vi "tcpGCS.vi"() -> ()   [LabVIEW 2014]
panel:
  in  "SRIC_PUSH":bool
  in  "SRIC_SSID":bool
  in  "Timer (s)":string="30"
  in  "Sync Config":bool
  in  "Password":string="pass"
  in  "Username":string="user"
  in  "Reconnect_Network":string="ubnt"
  in  "Delimiter":string="|"
  in  "File":string="msg.txt"
  in  "Directory":string="AC/"
  in  "IP Address":string="134.230.1.60"
  in  "ssid_key":string="74E87484EC"
  in  "sric_ssid":string="scrouter1"
  out "Config to Android":string
  in  "Ground Tranceiver Ip":string="192.168.1.20"
  in  "Air Tranceiver Ip":string="192.168.1.19"
  in  "Payload Ip":string="192.168.1.100"
  out "Acquiring Pictures":bool
  out "Unknown SRIC Message":string
  out "SRIC Message":string
  in  "SRIC":bool
  out "appended path":path
  out "Payload":bool
  out "Air Transceiver":bool
  out "Ground Transceiver":bool
  in  "Picture Interval":u8=3 format="%.0f seconds"
  in  "Set Picture Interval":bool
  out "connected 2":bool caption="connected"
  in  "wakeLock":bool
  in  "Rebalance":bool
  out "thing2":bool
  out "Average Time":dbl
  in  "ContinuousMode":bool
  out "thing1":bool
  out "ImageCount":u16
  out "unsigned byte array":u8[](array[numeric])
  out "Completed Images":u16[](array[numeric])
  out "OutputImages":T1(array[cluster])
  out "AverageTimePerMessage":dbl
  out "queue out":refnum<queue>
  in  "stop 2":bool
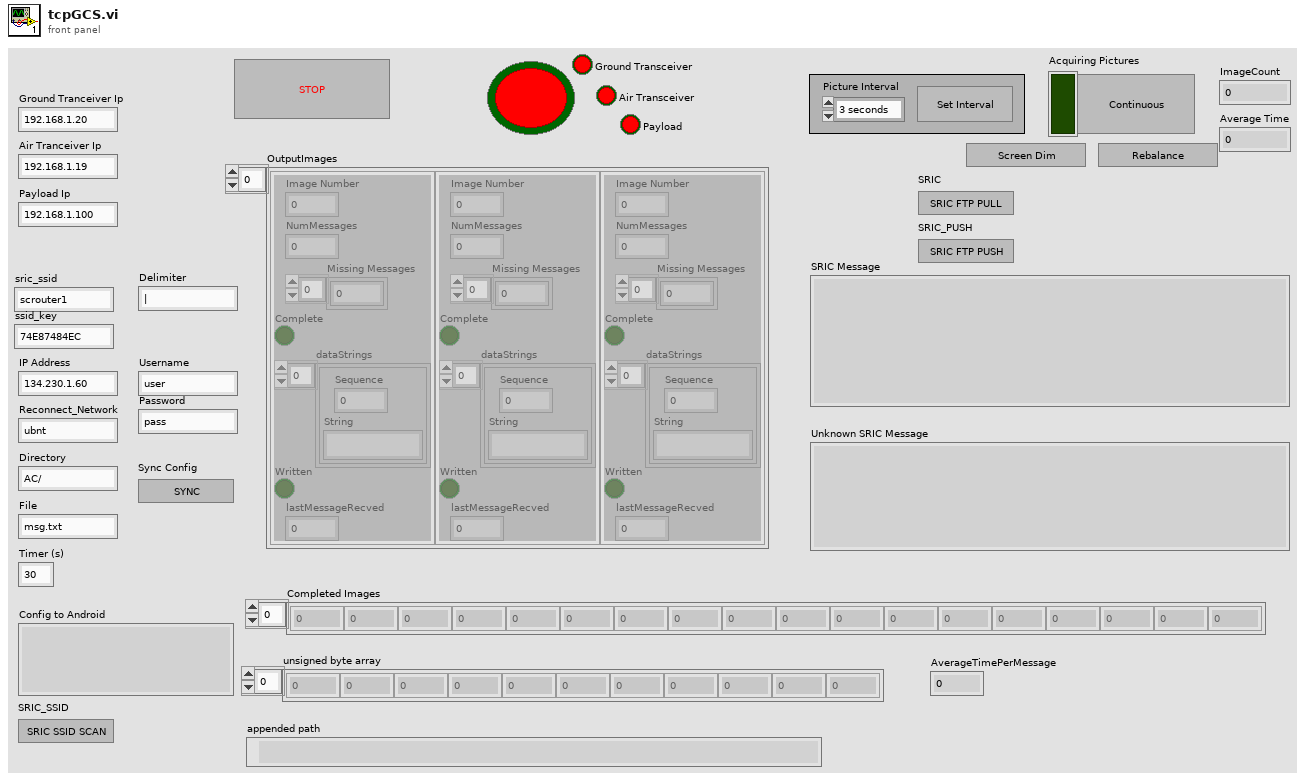
[diagram p1: front panel]
types:
  T1 = cluster{"Image Number":u16, "NumMessages":u16, "Missing Messages":u16[], "Complete":bool, "dataStrings":cluster{"Sequence":u16, "String":string}[], "Written":bool, "lastMessageRecved":u32}[]
  T2 = enum16{"Standard", "Buffered", "CRLF", "Immediate"}
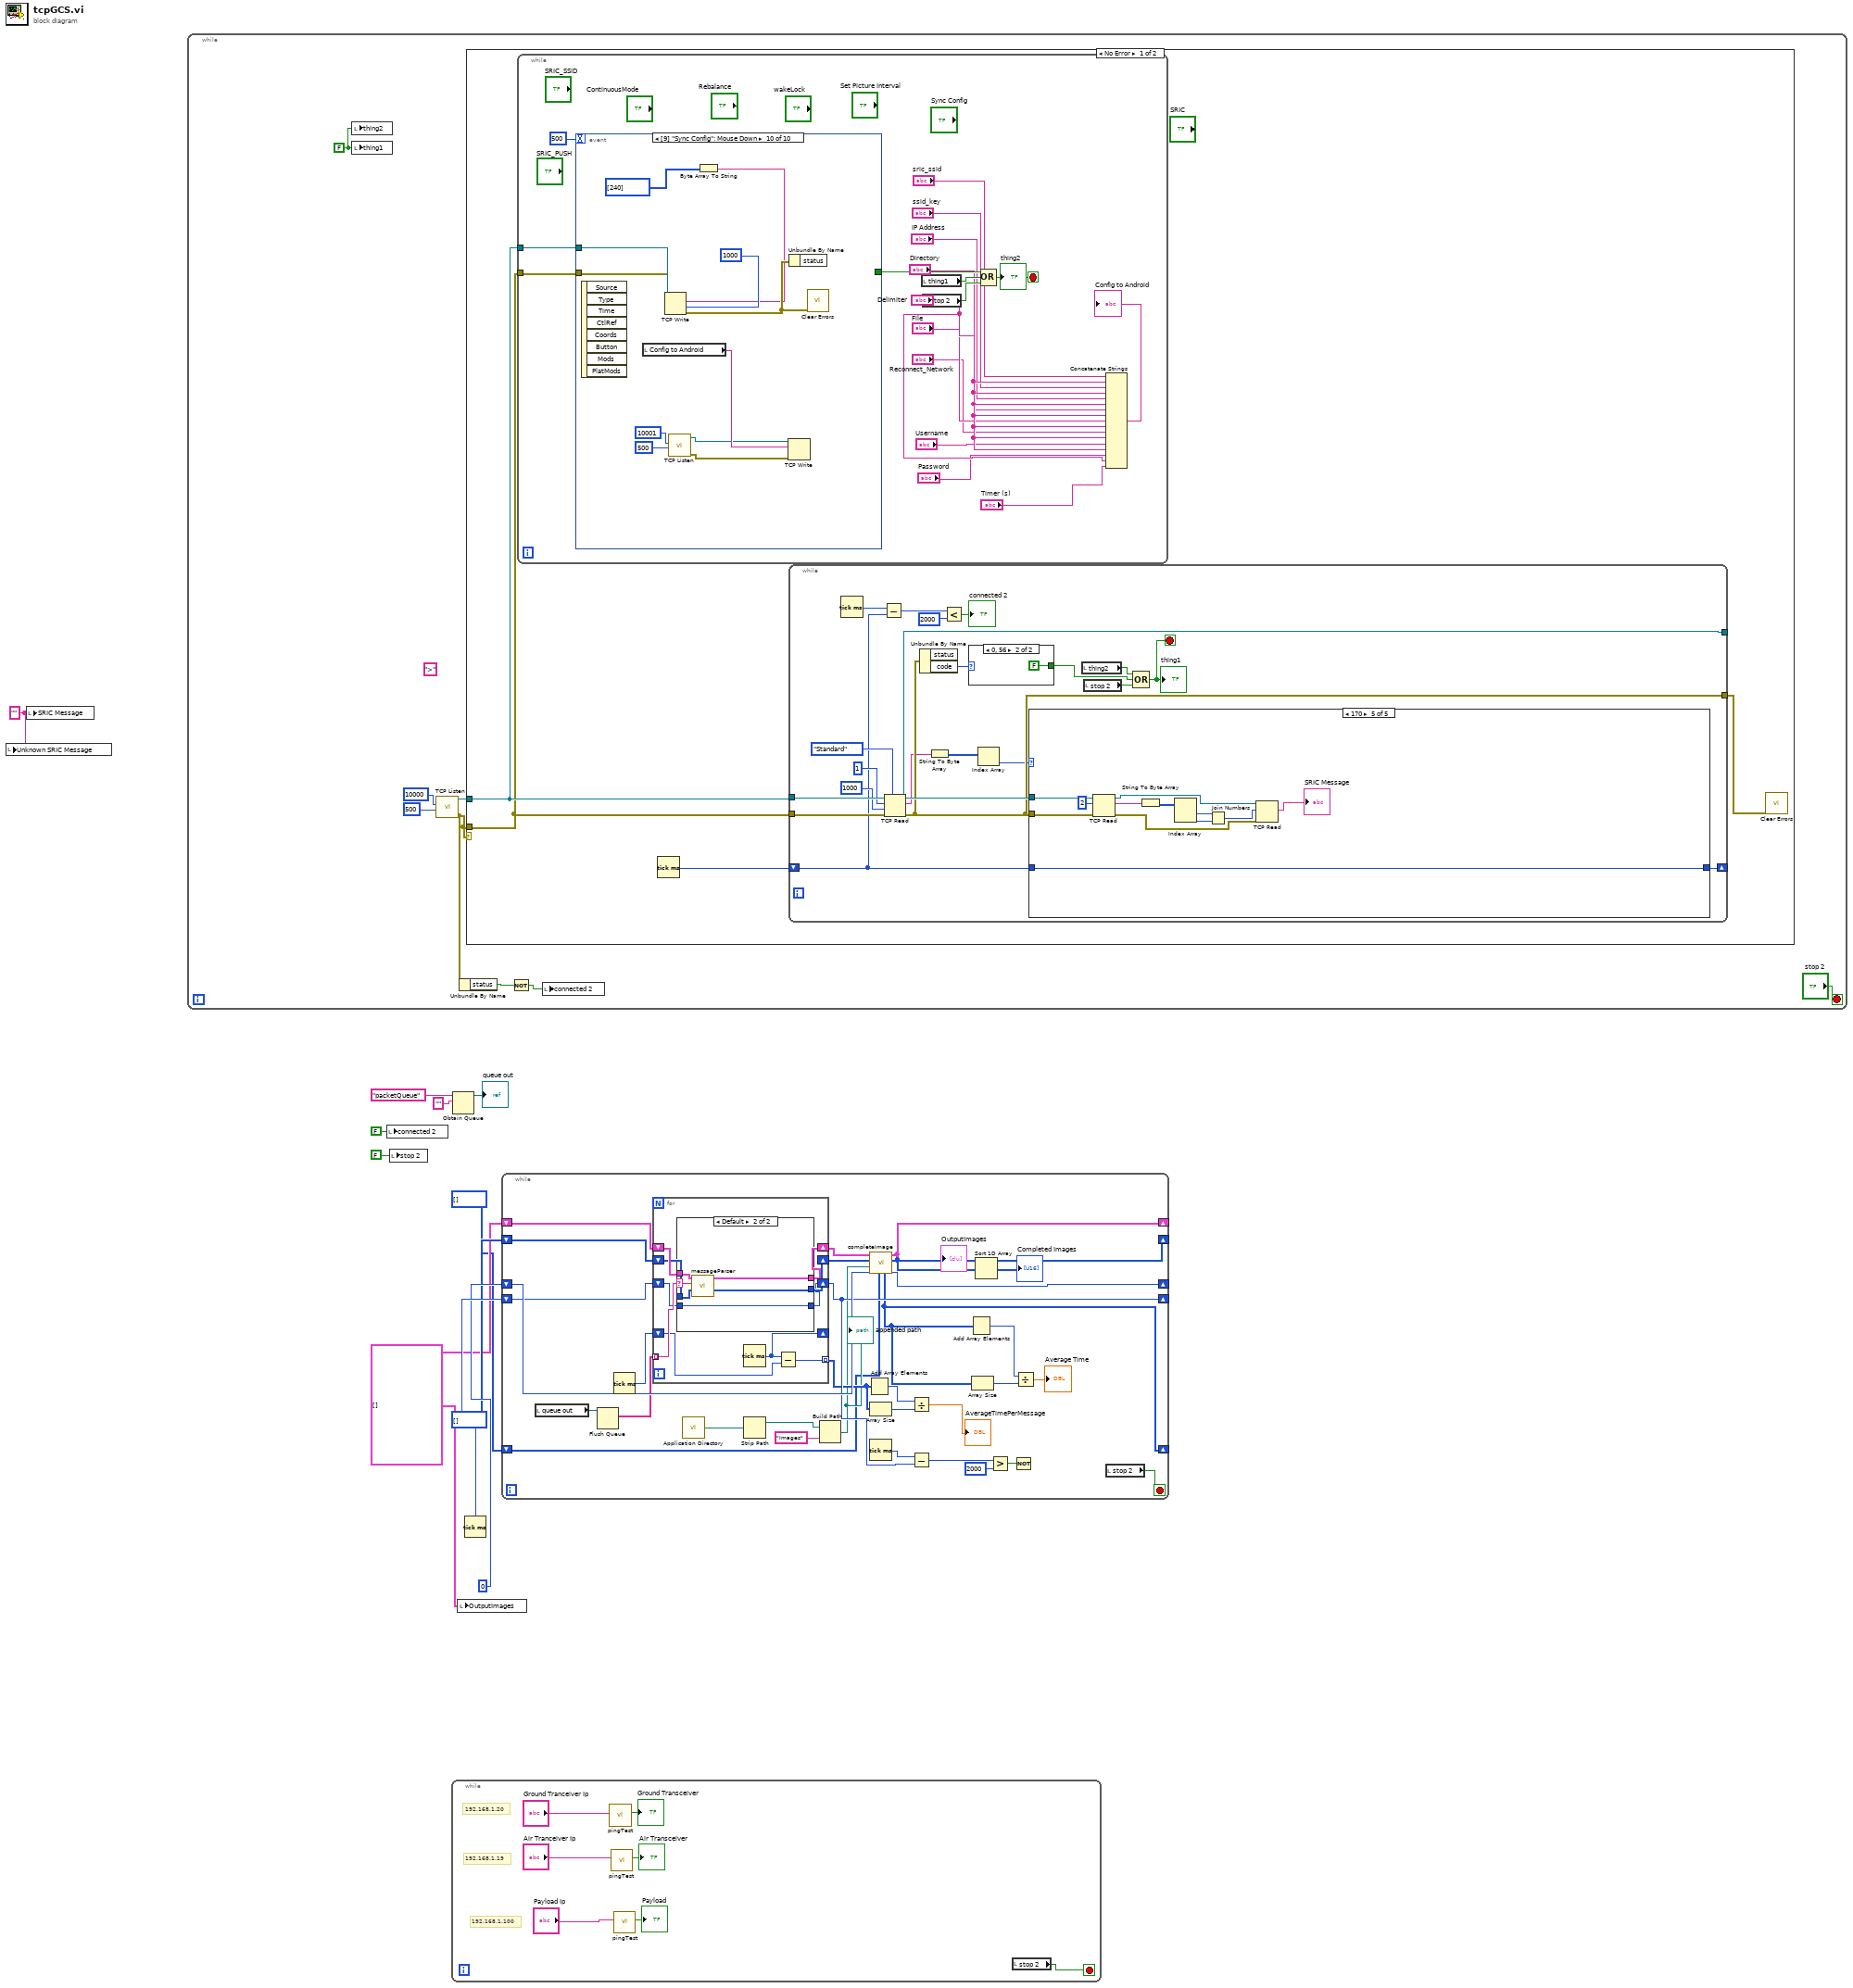
[diagram p0: block diagram]
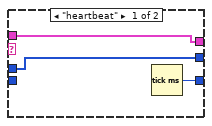
[diagram p2: hidden frame]
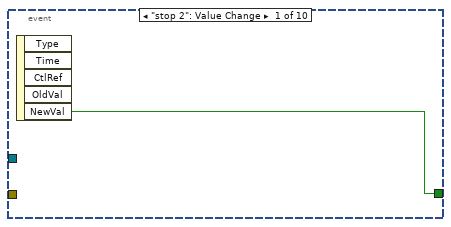
[diagram p3: hidden frame]
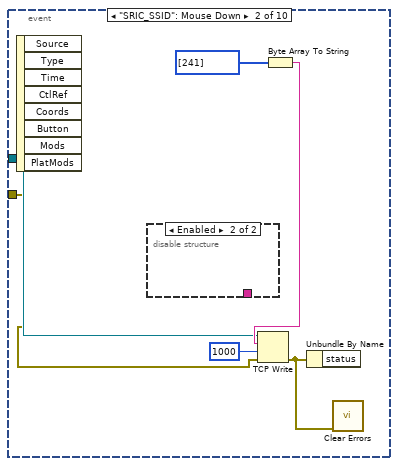
[diagram p4: hidden frame]
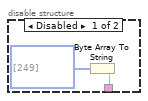
[diagram p5: hidden frame]
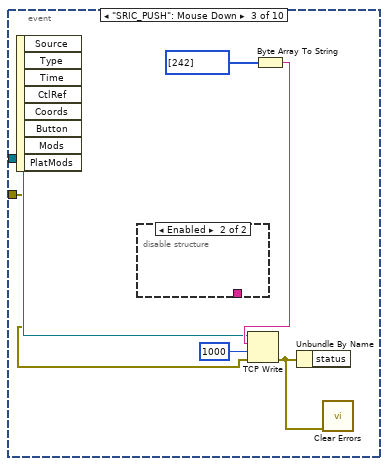
[diagram p6: hidden frame]
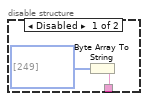
[diagram p7: hidden frame]
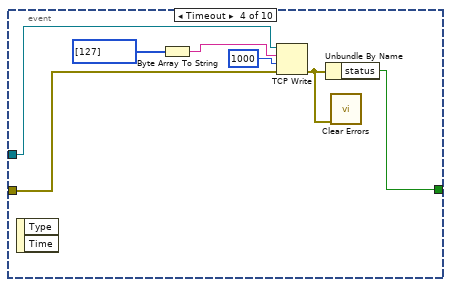
[diagram p8: hidden frame]
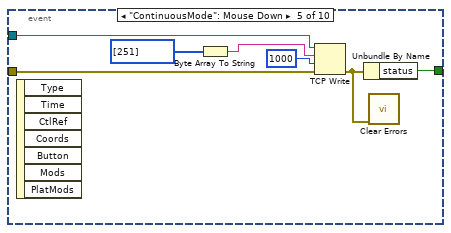
[diagram p9: hidden frame]
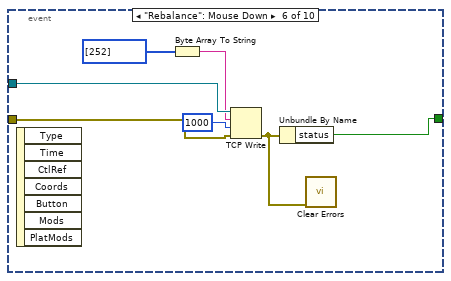
[diagram p10: hidden frame]
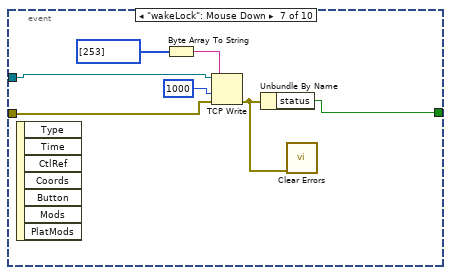
[diagram p11: hidden frame]
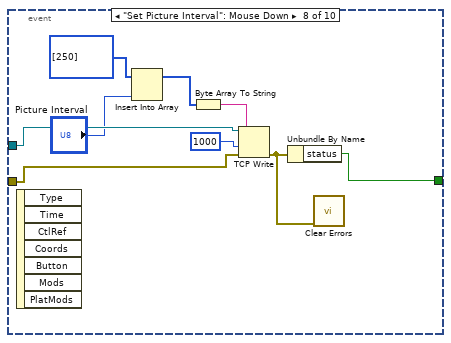
[diagram p12: hidden frame]
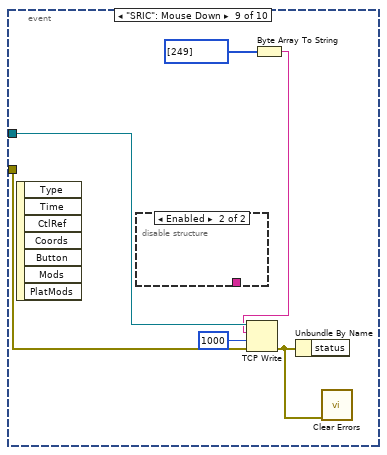
[diagram p13: hidden frame]
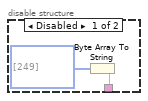
[diagram p14: hidden frame]
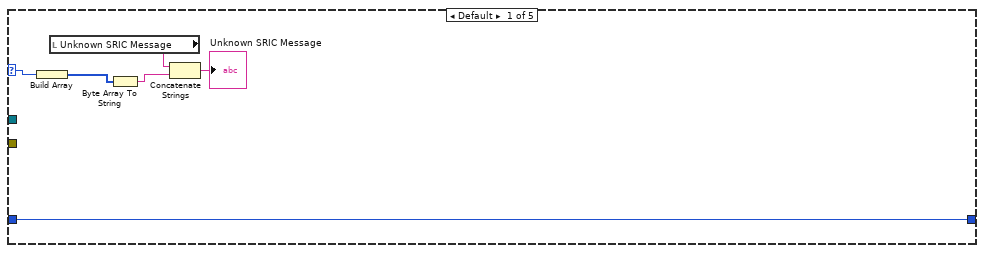
[diagram p15: hidden frame]
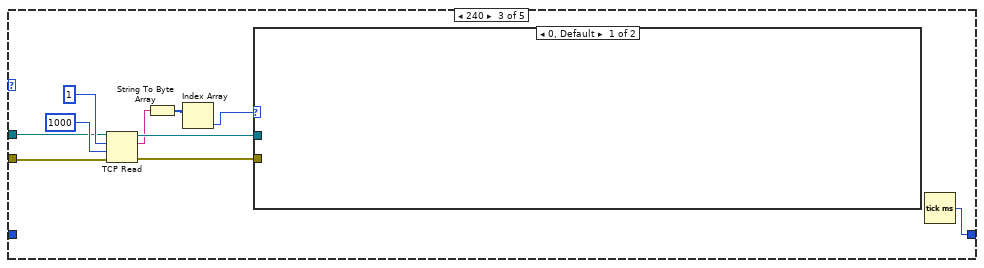
[diagram p17: hidden frame]
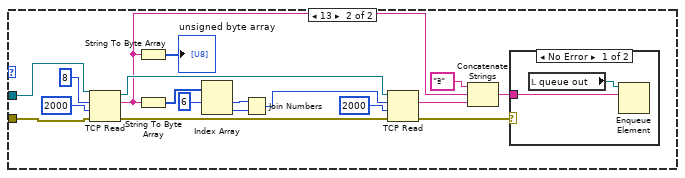
[diagram p18: hidden frame]
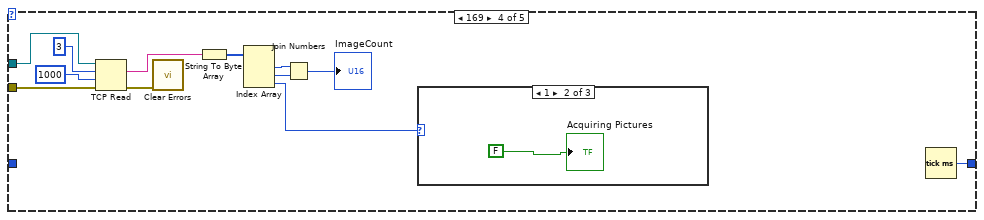
[diagram p20: hidden frame]
diagram:
  w1 = "" ("SRIC Message")
  w4 = T1 [] ("OutputImages 2")
  n1 = local write "Unknown SRIC Message"(w1) -> ()
  n2 = local write "SRIC Message"(w1) -> ()
  n3 = while {
    stop <- "stop 2" stop-if-true
    (unwired) ">" ("string")
    w15 = FALSE ("thing2")
    n4 = local write "thing2"(w15) -> ()
    n5 = local write "thing1"(w15) -> ()
    n6 = call <vilib>:"TCP Listen.vi"("timeout ms (wait forever: -1)"=500, "port"=u16 10000) -> ("error out"=w14:errorcluster, "connection ID"=w19:refnum<k5>)  [unwired: 5 in, 3 out]
    n7 = Unbundle By Name(w14) -> ("status"=w13:bool)
    n8 = case shown="No Error" w14 {
      tunnel: w19 -> [w23 _]
      tunnel: w14 -> [w22 _]
      frame No Error {
        n9 = while {
          tunnel: w23 -> [w37]
          tunnel: w22 -> [w36]
          stop <- w40 stop-if-true
          n10 = event shown="[9] \"Sync Config\": Mouse Down" {
            selector: _ -> [_ _ _ _ _ _ _ _ _ _]
            dyn-events: _ -> [_ _ _ _ _ _ _ _ _ _]
            timeout: 500 -> [_ _ _ _ _ _ _ _ _ _]
            tunnel: [w42 _ _ w59 w67 w78 w80 w90 _ _] -> w38
            tunnel: w37 -> [_ w44 w52 w61 w72 w77 w81 w93 w99 w112]
            tunnel: w36 -> [_ w43 w51 w60 w71 w76 w82 w92 w98 w111]
            event "stop 2": Value Change {
              n11 = event-data() -> ("NewVal"=w42:bool)  [unwired: 1 in, 4 out]
            }
            event "SRIC_SSID": Mouse Down {
              n12 = event-data() -> ()  [unwired: 1 in, 8 out]
              n13 = disable-structure shown="Enabled" {
                disable-tunnel: [w49 _] -> _
                frame Disabled {
                  n14 = Byte Array To String(unsigned byte array=u8[] [249]) -> (string=w49:string)
                }
                frame Enabled {
                }
              }
              n15 = Byte Array To String(unsigned byte array=u8[] [241]) -> (string=w48:string)
              n16 = TCP Write(connection ID=w44, data in=w48, error in (no error)=w43, 9:1000 ("timeout ms (25000)")) -> (error out=w46:errorcluster)  [unwired: 2 out]
              n17 = Unbundle By Name(w46) -> ()  [unwired: 1 out]
              n18 = call <vilib>:"Clear Errors.vi"("error in (no error)"=w46) -> ()  [unwired: 5 in, 2 out]
            }
            event "SRIC_PUSH": Mouse Down {
              n19 = event-data() -> ()  [unwired: 1 in, 8 out]
              n20 = disable-structure shown="Enabled" {
                disable-tunnel: [w57 _] -> _
                frame Disabled {
                  n21 = Byte Array To String(unsigned byte array=u8[] [249]) -> (string=w57:string)
                }
                frame Enabled {
                }
              }
              n22 = Byte Array To String(unsigned byte array=u8[] [242]) -> (string=w56:string)
              n23 = TCP Write(connection ID=w52, data in=w56, error in (no error)=w51, 9:1000 ("timeout ms (25000)")) -> (error out=w54:errorcluster)  [unwired: 2 out]
              n24 = Unbundle By Name(w54) -> ()  [unwired: 1 out]
              n25 = call <vilib>:"Clear Errors.vi"("error in (no error)"=w54) -> ()  [unwired: 5 in, 2 out]
            }
            event Timeout {
              n26 = event-data() -> ()  [unwired: 1 in, 2 out]
              n27 = Byte Array To String(unsigned byte array=u8[] [127]) -> (string=w65:string)
              n28 = TCP Write(connection ID=w61, data in=w65, error in (no error)=w60, 9:1000 ("timeout ms (25000)")) -> (error out=w62:errorcluster)  [unwired: 2 out]
              n29 = Unbundle By Name(w62) -> ("status"=w59:bool)
              n30 = call <vilib>:"Clear Errors.vi"("error in (no error)"=w62) -> ()  [unwired: 5 in, 2 out]
            }
            event "ContinuousMode": Mouse Down {
              n31 = event-data() -> ()  [unwired: 1 in, 7 out]
              n32 = Byte Array To String(unsigned byte array=u8[] [251]) -> (string=w70:string)
              n33 = TCP Write(connection ID=w72, data in=w70, error in (no error)=w71, 9:1000 ("timeout ms (25000)")) -> (error out=w66:errorcluster)  [unwired: 2 out]
              n34 = Unbundle By Name(w66) -> ("status"=w67:bool)
              n35 = call <vilib>:"Clear Errors.vi"("error in (no error)"=w66) -> ()  [unwired: 5 in, 2 out]
            }
            event "Rebalance": Mouse Down {
              n36 = event-data() -> ()  [unwired: 1 in, 7 out]
              n37 = Byte Array To String(unsigned byte array=u8[] [252]) -> (string=w74:string)
              n38 = TCP Write(connection ID=w77, data in=w74, error in (no error)=w76, 9:1000 ("timeout ms (25000)")) -> (error out=w73:errorcluster)  [unwired: 2 out]
              n39 = Unbundle By Name(w73) -> ("status"=w78:bool)
              n40 = call <vilib>:"Clear Errors.vi"("error in (no error)"=w73) -> ()  [unwired: 5 in, 2 out]
            }
            event "wakeLock": Mouse Down {
              n41 = event-data() -> ()  [unwired: 1 in, 7 out]
              n42 = Byte Array To String(unsigned byte array=u8[] [253]) -> (string=w84:string)
              n43 = TCP Write(connection ID=w81, data in=w84, error in (no error)=w82, 9:1000 ("timeout ms (25000)")) -> (error out=w83:errorcluster)  [unwired: 2 out]
              n44 = Unbundle By Name(w83) -> ("status"=w80:bool)
              n45 = call <vilib>:"Clear Errors.vi"("error in (no error)"=w83) -> ()  [unwired: 5 in, 2 out]
            }
            event "Set Picture Interval": Mouse Down {
              n46 = event-data() -> ()  [unwired: 1 in, 7 out]
              n47 = Insert Into Array(array=u8[] [250] ("unsigned byte array"), new element="Picture Interval") -> (w88:u8[])  [unwired: 1 in]
              n48 = Byte Array To String(unsigned byte array=w88) -> (string=w94:string)
              n49 = TCP Write(connection ID=w93, data in=w94, error in (no error)=w92, 9:1000 ("timeout ms (25000)")) -> (error out=w91:errorcluster)  [unwired: 2 out]
              n50 = Unbundle By Name(w91) -> ("status"=w90:bool)
              n51 = call <vilib>:"Clear Errors.vi"("error in (no error)"=w91) -> ()  [unwired: 5 in, 2 out]
            }
            event "SRIC": Mouse Down {
              n52 = event-data() -> ()  [unwired: 1 in, 7 out]
              n53 = disable-structure shown="Enabled" {
                disable-tunnel: [w102 _] -> _
                frame Disabled {
                  n54 = Byte Array To String(unsigned byte array=u8[] [249]) -> (string=w102:string)
                }
                frame Enabled {
                }
              }
              n55 = Byte Array To String(unsigned byte array=u8[] [249]) -> (string=w96:string)
              n56 = TCP Write(connection ID=w99, data in=w96, error in (no error)=w98, 9:1000 ("timeout ms (25000)")) -> (error out=w100:errorcluster)  [unwired: 2 out]
              n57 = Unbundle By Name(w100) -> ()  [unwired: 1 out]
              n58 = call <vilib>:"Clear Errors.vi"("error in (no error)"=w100) -> ()  [unwired: 5 in, 2 out]
            }
            event "Sync Config": Mouse Down {
              n59 = event-data() -> ()  [unwired: 1 in, 8 out]
              n60 = local read "Config to Android"() -> (w108:string)
              n61 = call <vilib>:"TCP Listen.vi"("timeout ms (wait forever: -1)"=500, "port"=u16 10001) -> ("error out"=w104:errorcluster, "connection ID"=w105:refnum<k5>)  [unwired: 5 in, 3 out]
              n62 = Byte Array To String(unsigned byte array=u8[] [240]) -> (string=w109:string)
              n63 = TCP Write(connection ID=w112, data in=w109, error in (no error)=w111, 9:1000 ("timeout ms (25000)")) -> (error out=w113:errorcluster)  [unwired: 2 out]
              n64 = TCP Write(connection ID=w105, data in=w108, error in (no error)=w104) -> ()  [unwired: 1 in, 3 out]
              n65 = Unbundle By Name(w113) -> ()  [unwired: 1 out]
              n66 = call <vilib>:"Clear Errors.vi"("error in (no error)"=w113) -> ()  [unwired: 5 in, 2 out]
            }
          }
          n67 = local read "thing1"() -> (w39:bool)
          n68 = local read "stop 2"() -> (w41:bool)
          n69 = Compound Arithmetic op=OR(w38, w39, w41) -> (w40:bool)
          "thing2" <- w40
          n70 = Concatenate Strings("sric_ssid", "Delimiter", "ssid_key", "Delimiter", "IP Address", "Delimiter", "Directory", "Delimiter", "File", "Delimiter", "Reconnect_Network", "Delimiter", "Username", "Delimiter", "Password", "Delimiter", "Timer (s)") -> (→"Config to Android":string)
        }
        n71 = Tick Count (ms)() -> (millisecond timer value=w21:u32)
        n72 = while {
          tunnel: w23 -> [w135]
          tunnel: w22 -> [w134]
          tunnel: [w126] -> _
          tunnel: [w125] -> w20
          shift-right: [w121] -> _
          shift-left: w21 -> [w116]
          stop <- w128 stop-if-true
          n73 = Tick Count (ms)() -> (millisecond timer value=w117:u32)
          n74 = Subtract(x=w117, y=w116) -> (x-y=w118:u32)
          n75 = TCP Read(connection ID=w135, bytes to read=1, error in (no error)=w134, 7:T2."Standard" ("mode (standard)"), 9:1000 ("timeout ms (25000)")) -> (connection ID out=w126:refnum<k5>, data out=w115:string, error out=w125:errorcluster)
          n76 = Unbundle By Name(w125) -> ("code"=w130:i32)  [unwired: 1 out]
          n77 = String To Byte Array(string=w115) -> (unsigned byte array=w124:u8[])
          n78 = Less?(x=w118, y=u32 2000) -> (x < y?=→"connected 2":bool)
          n79 = case shown="0, 56" w130 {
            tunnel: [TRUE FALSE] -> w129
            frame Default {
            }
            frame 0, 56 {
            }
          }
          n80 = Index Array(array=w124) -> (element=w123:u8)  [unwired: 1 in]
          n81 = case shown="170" w123 {
            selector: w123 -> [w140 _ _ _ _]
            tunnel: w126 -> [_ _ w150 w184 w197]
            tunnel: w125 -> [_ _ w149 w183 w196]
            tunnel: [w141 w142 w143 w174 w198] -> w121
            tunnel: w116 -> [w141 w142 _ _ w198]
            frame Default {
              n82 = Build Array(w140) -> (w139:u8[])
              n83 = local read "Unknown SRIC Message"() -> (w136:string)
              n84 = Byte Array To String(unsigned byte array=w139) -> (string=w138:string)
              n85 = Concatenate Strings(w136, w138) -> (→"Unknown SRIC Message":string)
            }
            frame 0 {
            }
            frame 240 {
              n86 = TCP Read(connection ID=w150, bytes to read=1, error in (no error)=w149, 9:1000 ("timeout ms (25000)")) -> (connection ID out=w148:refnum<k5>, data out=w145:string, error out=w147:errorcluster)  [unwired: 1 in]
              n87 = String To Byte Array(string=w145) -> (unsigned byte array=w146:u8[])
              n88 = Index Array(array=w146) -> (element=w144:u8)  [unwired: 1 in]
              n89 = case shown="0, Default" w144 {
                tunnel: w148 -> [_ w155]
                tunnel: w147 -> [_ w154]
                frame 0, Default {
                }
                frame 13 {
                  n90 = TCP Read(connection ID=w155, bytes to read=8, error in (no error)=w154, 9:2000 ("timeout ms (25000)")) -> (connection ID out=w165:refnum<k5>, data out=w159:string, error out=w164:errorcluster)  [unwired: 1 in]
                  n91 = String To Byte Array(string=w159) -> (unsigned byte array=→"unsigned byte array":u8[])
                  n92 = String To Byte Array(string=w159) -> (unsigned byte array=w169:u8[])
                  n93 = Index Array(array=w169, index #1=6 ("index")) -> (element #1=w167:u8, element #2=w166:u8)  [unwired: 1 in]
                  n94 = Join Numbers(hi=w167, lo=w166) -> ((hi.lo)=w153:u16)
                  n95 = TCP Read(connection ID=w165, bytes to read=w153, error in (no error)=w164, 9:2000 ("timeout ms (25000)")) -> (data out=w161:string, error out=w156:errorcluster)  [unwired: 1 in, 1 out]
                  n96 = Concatenate Strings("ª" ("y"), w159, w161) -> (w163:string)
                  n97 = case shown="No Error" w156 {
                    tunnel: w163 -> [w171 _]
                    frame No Error {
                      n98 = local read "queue out"() -> (w172:refnum<queue>)
                      n99 = Enqueue Element(queue=w172, element=w171) -> ()  [unwired: 2 in, 3 out]
                    }
                    frame Error {
                    }
                  }
                }
              }
              n100 = Tick Count (ms)() -> (millisecond timer value=w143:u32)
            }
            frame 169 {
              n101 = TCP Read(connection ID=w184, bytes to read=3, error in (no error)=w183, 9:1000 ("timeout ms (25000)")) -> (data out=w181:string, error out=w175:errorcluster)  [unwired: 1 in, 1 out]
              n102 = call <vilib>:"Clear Errors.vi"("error in (no error)"=w175) -> ()  [unwired: 5 in, 2 out]
              n103 = String To Byte Array(string=w181) -> (unsigned byte array=w180:u8[])
              n104 = Index Array(array=w180) -> (element #1=w179:u8, element #2=w178:u8, element #3=w173:u8)  [unwired: 3 in]
              n105 = Join Numbers(hi=w179, lo=w178) -> ((hi.lo)=→"ImageCount":u16)
              n106 = case shown="1" w173 {
                frame 0, Default {
                }
                frame 1 {
                  "Acquiring Pictures" <- FALSE ("Acquiring Pictures")
                }
                frame 15 {
                  n107 = local write "Acquiring Pictures"(TRUE ("Acquiring Pictures")) -> ()
                }
              }
              n108 = Tick Count (ms)() -> (millisecond timer value=w174:u32)
            }
            frame 170 {
              n109 = TCP Read(connection ID=w197, bytes to read=2, error in (no error)=w196) -> (connection ID out=w190:refnum<k5>, data out=w194:string, error out=w189:errorcluster)  [unwired: 2 in]
              n110 = String To Byte Array(string=w194) -> (unsigned byte array=w193:u8[])
              n111 = Index Array(array=w193) -> (element #1=w192:u8, element #2=w191:u8)  [unwired: 2 in]
              n112 = Join Numbers(hi=w192, lo=w191) -> ((hi.lo)=w188:u16)
              n113 = TCP Read(connection ID=w190, bytes to read=w188, error in (no error)=w189) -> (data out=→"SRIC Message":string)  [unwired: 2 in, 2 out]
            }
          }
          n114 = local read "thing2"() -> (w122:bool)
          n115 = local read "stop 2"() -> (w127:bool)
          n116 = Compound Arithmetic op=OR(w122, w129, w127) -> (w128:bool)
          "thing1" <- w128
        }
        n117 = call <vilib>:"Clear Errors.vi"("error in (no error)"=w20) -> ()  [unwired: 5 in, 2 out]
      }
      frame Error {
      }
    }
    n118 = Not(x=w13) -> (.not. x?=w12:bool)
    n119 = local write "connected 2"(w12) -> ()
  }
  n120 = local write "connected 2"(FALSE ("connected")) -> ()
  n121 = local write "stop 2"(FALSE ("stop 2")) -> ()
  n122 = while {
    stop <- w207 stop-if-true
    # "192.168.1.100"
    # "192.168.1.19"
    # "192.168.1.20"
    n123 = call "pingTest.vi"("IpAddress"="Ground Tranceiver Ip") -> ("Available"=→"Ground Transceiver":bool)  [unwired: 10 in]
    n124 = call "pingTest.vi"("IpAddress"="Air Tranceiver Ip") -> ("Available"=→"Air Transceiver":bool)  [unwired: 10 in]
    n125 = call "pingTest.vi"("IpAddress"="Payload Ip") -> ("Available"=→"Payload":bool)  [unwired: 10 in]
    n126 = local read "stop 2"() -> (w207:bool)
  }
  n127 = Obtain Queue(name (unnamed)="packetQueue", element data type="") -> (queue out=→"queue out":refnum<queue>)  [unwired: 3 in, 2 out]
  n128 = local write "OutputImages"(w4) -> ()
  n129 = Tick Count (ms)() -> (millisecond timer value=w7:u32)
  n130 = while {
    shift-right: [w234] -> _
    shift-left: w4 -> [w238]
    shift-right: [w236] -> _
    shift-left: u16[] [] ("Array 2") -> [w237]
    shift-right: [w230] -> _
    shift-left: 0 ("Numeric 2") -> [w231]
    shift-right: [w227] -> _
    shift-left: w7 -> [w229]
    shift-right: [w212] -> _
    shift-left: u32[] [] ("Times Out") -> [w213]
    stop <- w239 stop-if-true
    n131 = local read "queue out"() -> (w218:refnum<queue>)
    n132 = Flush Queue(queue=w218) -> (remaining elements=w217:string[])  [unwired: 1 in, 2 out]
    n133 = Tick Count (ms)() -> (millisecond timer value=w223:u32)
    n134 = for {
      shift-right: [w248] -> w233
      shift-left: w238 -> [w249]
      shift-right: [w246] -> w232
      shift-left: w237 -> [w247]
      tunnel: w217 -> [w245] mode=indexing
      shift-right: [w244] -> w227
      shift-left: w229 -> [w243]
      shift-right: [w242] -> _
      shift-left: w223 -> [w241]
      tunnel: [w240] -> w222 mode=indexing
      n135 = case shown="Default" w245 {
        selector: w245 -> [_ w254]
        tunnel: w249 -> [w252 w258]
        tunnel: [w252 w257] -> w248
        tunnel: w247 -> [w251 w256]
        tunnel: [w251 w255] -> w246
        tunnel: [w250 w253] -> w244
        tunnel: w243 -> [_ w253]
        frame "heartbeat" {
          n136 = Tick Count (ms)() -> (millisecond timer value=w250:u32)
        }
        frame Default {
          n137 = call "messageParser.vi"("Completed Images In"=w256, "Input"=w254, "Input Images"=w258) -> ("Completed Images Out"=w255:u16[], "OutputImages"=w257:T1)  [unwired: 7 in]
        }
      }
      n138 = Tick Count (ms)() -> (millisecond timer value=w242:u32)
      n139 = Subtract(x=w242, y=w241) -> (x-y=w240:u32)
    }
    n140 = call <vilib>:"Application Directory.vi"() -> ("Application Directory"=w208:path)
    n141 = Strip Path(path=w208) -> (stripped path=w216:path)  [unwired: 1 out]
    n142 = Build Path(base path=w216, name or relative path="Images") -> (appended path=w214:path)
    "appended path" <- w214
    n143 = Add Array Elements(numeric array=w222) -> (sum=w221:u32)
    n144 = call "completeImage.vi"("Times In"=w213, "Numeric"=w231, "file (use dialog)"=w214, "Array"=w232, "InputImages"=w233) -> ("Numeric 2"=w230:i32, "Array 2"=w236:u16[], "OutputImages"=w234:T1, "Times Out"=w212:u32[])  [unwired: 3 in]
    "OutputImages" <- w234
    n145 = Array Size(array=w222) -> (size(s)=w220:i32)
    n146 = Tick Count (ms)() -> (millisecond timer value=w228:u32)
    n147 = Divide(x=w221, y=w220) -> (x/y=→"AverageTimePerMessage":dbl)
    n148 = Subtract(x=w228, y=w227) -> (x-y=w226:u32)
    n149 = Add Array Elements(numeric array=w212) -> (sum=w211:u32)
    n150 = Array Size(array=w212) -> (size(s)=w210:i32)
    n151 = Sort 1D Array(array=w236) -> (sorted array=→"Completed Images":u16[])
    n152 = Greater?(x=w226, y=u32 2000) -> (0:w224:bool)
    n153 = Not(x=w224) -> ()  [unwired: 1 out]
    n154 = Divide(x=w211, y=w210) -> (x/y=→"Average Time":dbl)
    n155 = local read "stop 2"() -> (w239:bool)
  }
